vi "AutoMultiBall.vi"(8 "error in (no error)":errorcluster, 9 "Hot?":bool, 10 "Camera?":bool, 11 "ShotCount":u8=2) -> (0 "error out":errorcluster)   [LabVIEW 2013]
uses:
  AutoMultiBallStates.ctl
  ShooterStates.ctl
  <vilib>/Rock Robotics/WPI/Solenoid/WPI_SolenoidSetEnum.vi
  <vilib>/Rock Robotics/WPI/Solenoid/WPI_SolenoidValue.ctl
  Robot Global Data.vi
  ShooterCmds.ctl
  Position Typedef.ctl
panel:
  in  "Angle to Turn":dbl=15.0 format="%#_13g"
  in  "Not Hot Delay":u32=4000
  in  "Speed":dbl=0.75
  in  "Angle":dbl
  in  "Distance":dbl=84.0
  in  "Transfer Timeout (ms)":u32=1000
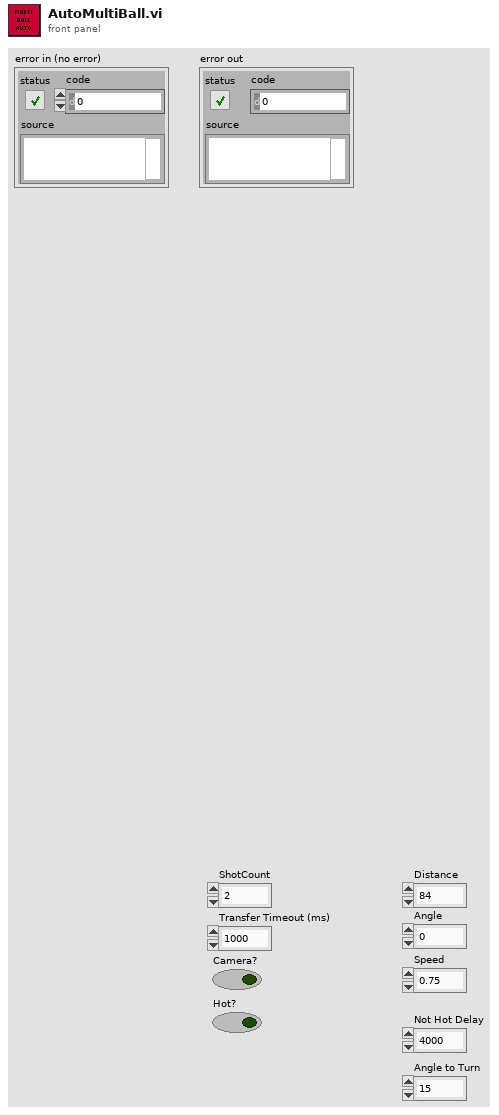
[diagram p1: front panel]
types:
  T1 = typedef "AutoMultiBallStates.ctl" = enum16{"Setup", "Wait To Fire", "Not Hot Delay", "Fire", "Pickup", "Transfer", "Cleanup"}
  T2 = typedef "WPI_SolenoidDevRef.ctl" = cluster{"DevStatus":errorcluster, "Solenoid Module":T3, "Forward Solenoid Channel":T4, "Reverse Solenoid Channel":T4}
  T3 = typedef "FPGA_TypedefSolenoidModule.ctl" = enum16{"Solenoid Module 1", "Solenoid Module 2"}
  T4 = typedef "WPI_SolenoidChannel.ctl" = enum8{"Solenoid 1", "Solenoid 2", "Solenoid 3", "Solenoid 4", "Solenoid 5", "Solenoid 6", "Solenoid 7", "Solenoid 8", "Invalid"}
  T5 = typedef "Position Typedef.ctl" = cluster{"X":dbl, "Y":dbl, "Heading":dbl}
  T6 = typedef "WPI_SolenoidValue.ctl" = enum16{"Off", "On", "Forward", "Reverse"}
  T7 = typedef "ShooterCmds.ctl" = enum16{"Fire", "Lob", "Retract", "End Of Match", "Release", "FireAuto"}
  T8 = typedef "ShooterStates.ctl" = enum16{"Init", "Ready", "RetractFull", "Disengage Clutch", "Clutch Delay", "Fire", "Fire Delay", "Latch", "Retract", "Release"}
  T9 = typedef "WPI_MotorControlDeviceRef.ctl" = cluster{"DeviceStatus":errorcluster, "Type":enum16{"PWM", "CAN"}, "PWM":cluster{"Digital Module":T10, "PWM Channel":T11, "DeadBand":T12}, "CAN":cluster{"Device Number":u8, "Control Mode":T13, "Semaphore":T14, "Max Vout":dbl}, "Invert":bool, "TransformRef":T15, "InvTransformRef":T15}
  T10 = typedef "FPGA_TypedefDigitalModule.ctl" = enum16{"Digital Module 1", "Digital Module 2"}
  T11 = typedef "FPGA_DIOPWMChannel.ctl" = enum8{"PWM 1", "PWM 2", "PWM 3", "PWM 4", "PWM 5", "PWM 6", "PWM 7", "PWM 8", "PWM 9", "PWM 10", "Invalid"}
  T12 = typedef "WPI_PWMDeadband.ctl" = cluster{"Name":string, "maxPositivePwm":i32, "minPositivePwm":i32, "centerPwm":i32, "maxNegativePwm":i32, "minNegativePwm":i32, "angularRange":u16}
  T13 = typedef "WPI_CANJaguar_ControlMode.ctl" = enum8{"Percent VBus", "Current", "Speed", "Position", "Voltage"}
  T14 = typedef "Semaphore RefNum" = refnum<k1>
  T15 = typedef "WPI_PWMTransform_ConPane.ctl" = refnum<vi>
  T16 = typedef "WPI_DigitalInputDevRef.ctl" = cluster{"DevStatus":errorcluster, "DIO Channel":T17, "Digital Module":T10}
  T17 = typedef "FPGA_DIOChannel.ctl" = enum8{"DIO 1", "DIO 2", "DIO 3", "DIO 4", "DIO 5", "DIO 6", "DIO 7", "DIO 8", "DIO 9", "DIO 10", "DIO 11", "DIO 12", "DIO 13", "DIO 14", "Invalid"}
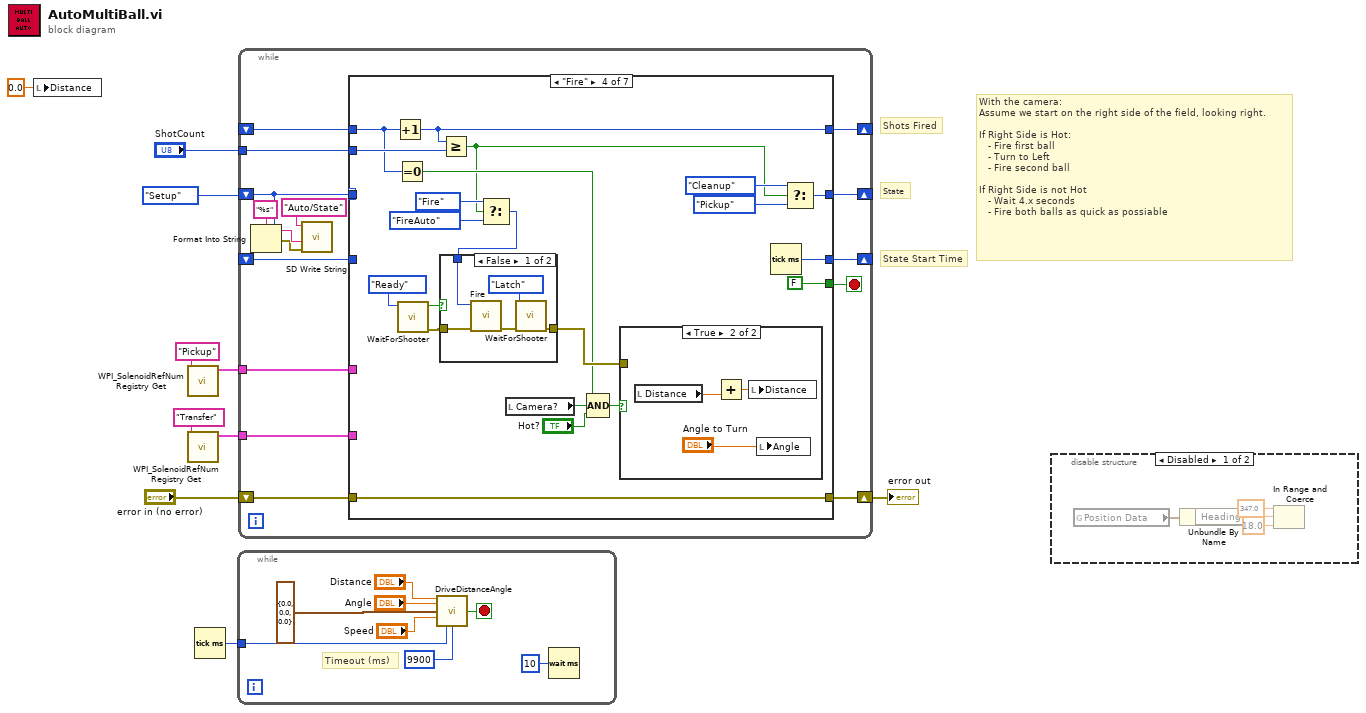
[diagram p0: block diagram]
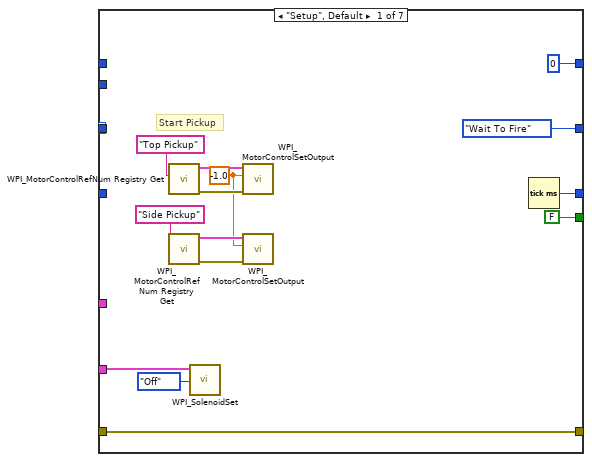
[diagram p3: hidden frame]
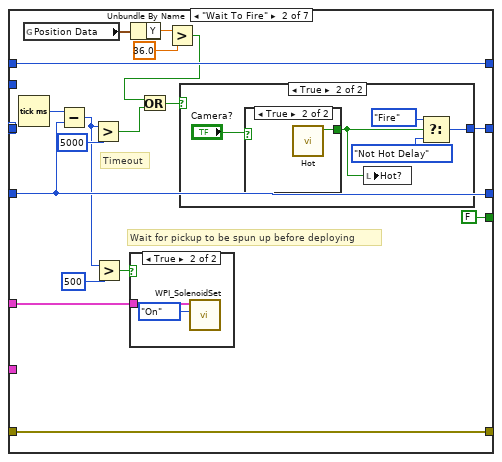
[diagram p4: hidden frame]
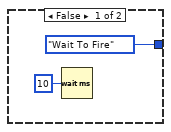
[diagram p6: hidden frame]
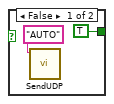
[diagram p7: hidden frame]
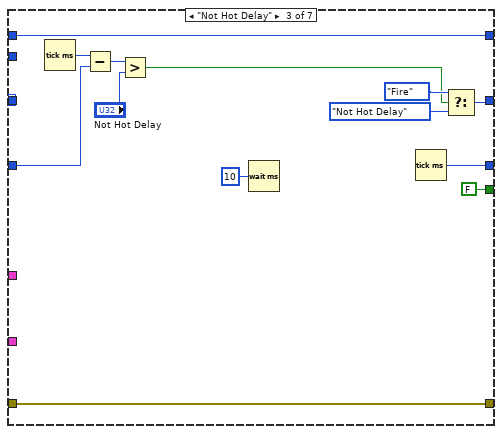
[diagram p8: hidden frame]
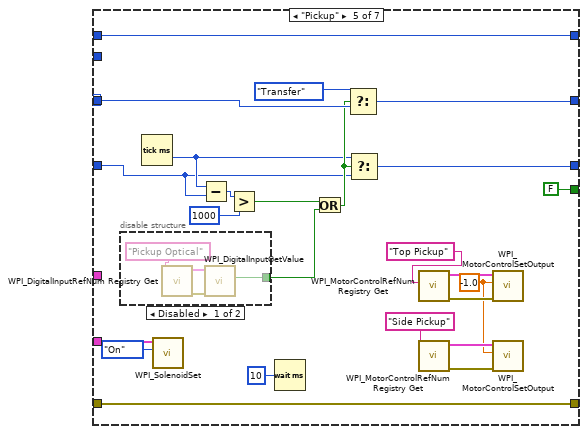
[diagram p11: hidden frame]
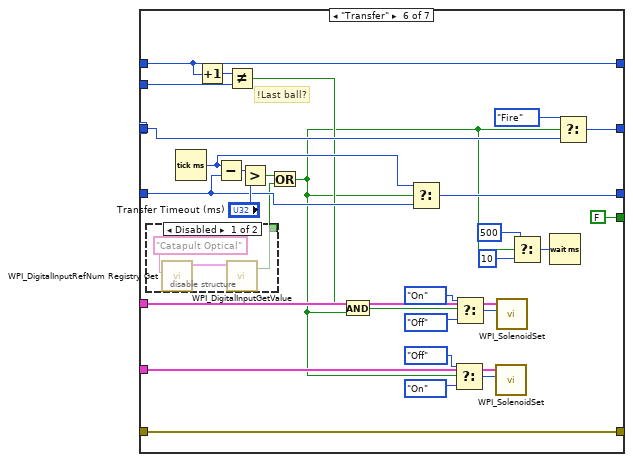
[diagram p13: hidden frame]
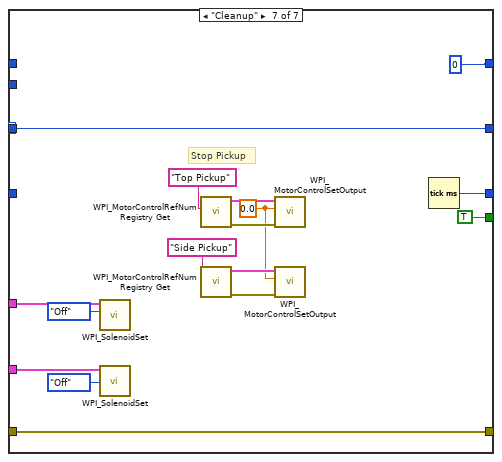
[diagram p15: hidden frame]
diagram:
  # "With the camera:\nAssume we start on the right side of the field, looking right.\n\nIf Right Side is Hot:\n   - Fire first ball\n   - Turn to Left \n   - Fire second ball\n\nIf Right Side is not Hot\n   - Wait 4.x seconds\n   - Fire both balls as quick as possiable"
  # "State Start Time"
  # "State"
  # "Shots Fired"
  n1 = local write "Distance"(0.0 ("X Target")) -> ()
  n2 = call <vilib>:"WPI_SolenoidRefNum Registry Get.vi"("refnum name"="Pickup") -> ("SolenoidDevRef"=w6:T2)  [unwired: 9 in, 1 out]
  n3 = call <vilib>:"WPI_SolenoidRefNum Registry Get.vi"("refnum name"="Transfer") -> ("SolenoidDevRef"=w4:T2)  [unwired: 9 in, 1 out]
  n4 = Tick Count (ms)() -> (millisecond timer value=w1:u32)
  n5 = while {
    tunnel: w1 -> [w17]
    stop <- w15 stop-if-true
    # "Timeout (ms)"
    n6 = call "DriveDistanceAngle.vi"("Distance"="Distance", "Angle"="Angle", "Starting Position"=T5 {"X"=0.0, "Y"=0.0, "Heading"=0.0}, "Speed"="Speed", "Start time"=w17, "Timeout (ms)"=u32 9900 ("y")) -> ("Timeout?"=w15:bool)  [unwired: 6 in, 3 out]
    n7 = Wait (ms)(milliseconds to wait=u32 10) -> ()  [unwired: 1 out]
  }
  n8 = while {
    shift-right: [w33] -> w3
    shift-left: "error in (no error)" -> [w34]
    shift-right: [w31] -> _
    shift-left: _ -> [w32]
    shift-right: [w29] -> _
    shift-left: AutoMultiBallStates."Setup" -> [w19]
    shift-right: [w27] -> _
    shift-left: _ -> [w28]
    tunnel: "ShotCount" -> [w26]
    tunnel: w6 -> [w25]
    tunnel: w4 -> [w24]
    stop <- w30 stop-if-true
    n9 = Format Into String(format string="%s", w19) -> (resulting string=w22:string, error out=w21:errorcluster)  [unwired: 2 in]
    n10 = call <vilib>:"SD Write String.vi"("error in"=w21, "String"=w22, "Name"="Auto/State") -> ()  [unwired: 7 in, 2 out]
    n11 = case shown="\"Fire\"" w19 {
      selector: w19 -> [_ _ _ _ w144 w177 _]
      tunnel: w34 -> [w35 w65 w88 w111 w142 w176 w183]
      tunnel: [w35 w65 w88 w111 w142 w176 w183] -> w33
      tunnel: [AutoMultiBallStates."Wait To Fire" w59 w79 w104 w143 w172 w182] -> w29
      tunnel: w32 -> [_ w56 w78 _ w135 w164 _]
      tunnel: [w47 w56 w87 w109 w145 w166 w196] -> w31
      tunnel: [FALSE ("At Target") FALSE ("At Target") FALSE ("At Target") FALSE FALSE FALSE ("At Target") TRUE ("At Target")] -> w30
      tunnel: w19 -> [_ _ _ _ _ _ w182]
      tunnel: w28 -> [_ w64 w90 w97 w139 w158 _]
      tunnel: [u8 0 ("ShotCount") w64 w90 w105 w139 w158 u8 0 ("ShotCount")] -> w27
      tunnel: w26 -> [_ _ _ w106 _ w156 _]
      tunnel: w25 -> [_ w58 _ _ _ w160 w193]
      tunnel: w24 -> [w37 _ _ _ w123 w168 w185]
      frame "Setup", Default {
        w38 = -1.0 ("Output")
        # "Start Pickup"
        n12 = call <vilib>:"WPI_MotorControlRefNum Registry Get.vi"("refnum name"="Top Pickup") -> ("error out"=w41:errorcluster, "MotorControlDevRef"=w45:T9)  [unwired: 9 in]
        n13 = call <vilib>:"WPI_MotorControlRefNum Registry Get.vi"("refnum name"="Side Pickup") -> ("error out"=w43:errorcluster, "MotorControlDevRef"=w42:T9)  [unwired: 9 in]
        n14 = call-poly <vilib>:"WPI_SolenoidSet.vi"("Value"=WPI_SolenoidValue."Off", "SolenoidDevRef"=w37) -> ()  [unwired: 8 in, 2 out]
        n15 = call <vilib>:"WPI_MotorControlSetOutput.vi"("error in (no error)"=w41, "Output"=w38, "MotorControlDevRef"=w45) -> ()  [unwired: 6 in, 3 out]
        n16 = call <vilib>:"WPI_MotorControlSetOutput.vi"("error in (no error)"=w43, "Output"=w38, "MotorControlDevRef"=w42) -> ()  [unwired: 6 in, 3 out]
        n17 = Tick Count (ms)() -> (millisecond timer value=w47:u32)
      }
      frame "Wait To Fire" {
        # "Timeout"
        # "Wait for pickup to be spun up before deploying"
        n18 = Tick Count (ms)() -> (millisecond timer value=w57:u32)
        n19 = global read "Robot Global Data.vi" "Position Data"() -> (w62:T5)
        n20 = Subtract(x=w57, y=w56) -> (x-y=w52:u32)
        n21 = Greater?(x=w52, y=u32 5000) -> (0:w49:bool)
        n22 = Greater?(x=w52, y=u32 500) -> (0:w54:bool)
        n23 = case shown="True" w54 {
          tunnel: w58 -> [_ w66]
          frame False {
          }
          frame True {
            n24 = call-poly <vilib>:"WPI_SolenoidSet.vi"("Value"=WPI_SolenoidValue."On", "SolenoidDevRef"=w66) -> ()  [unwired: 8 in, 2 out]
          }
        }
        n25 = Unbundle By Name(w62) -> ("Y"=w61:dbl)
        n26 = Greater?(x=w61, y=36.0) -> (0:w50:bool)
        n27 = Or(x=w50, y=w49) -> (x .or. y?=w51:bool)
        n28 = case shown="True" w51 {
          tunnel: [AutoMultiBallStates."Wait To Fire" ("f") w71] -> w59
          frame False {
            n29 = Wait (ms)(milliseconds to wait=u32 10) -> ()  [unwired: 1 out]
          }
          frame True {
            n30 = case shown="True" "Camera?" {
              tunnel: [TRUE ("Hot?") w77] -> w73
              frame False {
                n31 = call "SendUDP.vi"("data in"="AUTO") -> ()  [unwired: 10 in, 1 out]
              }
              frame True {
                n32 = call "Hot.vi"() -> ("Hot?"=w77:bool)  [unwired: 8 in, 3 out]
              }
            }
            n33 = local write "Hot?"(w73) -> ()
            n34 = Select(t=AutoMultiBallStates."Fire", s=w73, f=AutoMultiBallStates."Not Hot Delay") -> (s? t:f=w71:T1)
          }
        }
      }
      frame "Not Hot Delay" {
        n35 = Tick Count (ms)() -> (millisecond timer value=w85:u32)
        n36 = Subtract(x=w85, y=w78) -> (x-y=w84:u32)
        n37 = Greater?(x=w84, y="Not Hot Delay") -> (0:w80:bool)
        n38 = Wait (ms)(milliseconds to wait=u32 10) -> ()  [unwired: 1 out]
        n39 = Tick Count (ms)() -> (millisecond timer value=w87:u32)
        n40 = Select(t=AutoMultiBallStates."Fire", s=w80, f=AutoMultiBallStates."Not Hot Delay") -> (s? t:f=w79:T1)
      }
      frame "Fire" {
        n41 = Increment(x=w97) -> (x+1=w105:u8)
        n42 = Equal To 0?(x=w97) -> (x = 0?=w96:bool)
        n43 = call "WaitForShooter.vi"("State"=ShooterStates."Ready") -> ("error out"=w103:errorcluster, "Timeout"=w101:bool)  [unwired: 9 in]
        n44 = Greater Or Equal?(x=w105, y=w106) -> (x >= y?=w93:bool)
        n45 = Select(t=ShooterCmds."Fire", s=w93, f=ShooterCmds."FireAuto") -> (s? t:f=w92:T7)
        n46 = case shown="False" w101 {
          tunnel: w103 -> [w118 w121]
          tunnel: [w117 w121] -> w98
          tunnel: w92 -> [w116 _]
          frame False {
            n47 = call "Fire.vi"("error in (no error)"=w118, 11:w116) -> ("error out"=w119:errorcluster)  [unwired: 9 in]
            n48 = call "WaitForShooter.vi"("error in (no error)"=w119, "State"=ShooterStates."Latch") -> ("error out"=w117:errorcluster)  [unwired: 8 in, 1 out]
          }
          frame True {
          }
        }
        n49 = local read "Camera?"() -> (w100:bool)
        n50 = Compound Arithmetic op=AND(w96, w100, "Hot?") -> (w99:bool)
        n51 = case shown="True" w99 {
          tunnel: w98 -> [_ _]
          frame False {
          }
          frame True {
            n52 = local read "Distance"() -> (w115:dbl)
            n53 = Add(y=w115) -> (x=w113:dbl, x+y=w114:dbl)
            n54 = local write "Distance"(w114) -> ()
            n55 = local write "Angle"("Angle to Turn") -> ()
          }
        }
        n56 = Tick Count (ms)() -> (millisecond timer value=w109:u32)
        n57 = Select(t=AutoMultiBallStates."Cleanup", s=w93, f=AutoMultiBallStates."Pickup") -> (s? t:f=w104:T1)
      }
      frame "Pickup" {
        w124 = -1.0 ("Output")
        n58 = disable-structure shown="Disabled" {
          disable-tunnel: [w146 _] -> w138
          frame Disabled {
            n59 = call <vilib>:"WPI_DigitalInputRefNum Registry Get.vi"("refnum name"="Pickup Optical") -> ("error out"=w148:errorcluster, "DigitalInputDevRef"=w147:T16)  [unwired: 9 in]
            n60 = call <vilib>:"WPI_DigitalInputGetValue.vi"("error in (no error)"=w148, "DigitalInputDevRef"=w147) -> ("Value"=w146:bool)  [unwired: 7 in, 2 out]
          }
          frame Enabled {
          }
        }
        n61 = Tick Count (ms)() -> (millisecond timer value=w136:u32)
        n62 = call-poly <vilib>:"WPI_SolenoidSet.vi"("Value"=WPI_SolenoidValue."On", "SolenoidDevRef"=w123) -> ()  [unwired: 8 in, 2 out]
        n63 = Subtract(x=w136, y=w135) -> (x-y=w134:u32)
        n64 = Greater?(x=w134, y=u32 1000) -> (0:w132:bool)
        n65 = Wait (ms)(milliseconds to wait=u32 10) -> ()  [unwired: 1 out]
        n66 = Or(x=w132, y=w138) -> (x .or. y?=w137:bool)
        n67 = Select(t=AutoMultiBallStates."Transfer", s=w137, f=w144) -> (s? t:f=w143:T1)
        n68 = Select(t=w136, s=w137, f=w135) -> (s? t:f=w145:u32)
        n69 = call <vilib>:"WPI_MotorControlRefNum Registry Get.vi"("refnum name"="Top Pickup") -> ("error out"=w126:errorcluster, "MotorControlDevRef"=w130:T9)  [unwired: 9 in]
        n70 = call <vilib>:"WPI_MotorControlRefNum Registry Get.vi"("refnum name"="Side Pickup") -> ("error out"=w128:errorcluster, "MotorControlDevRef"=w127:T9)  [unwired: 9 in]
        n71 = call <vilib>:"WPI_MotorControlSetOutput.vi"("error in (no error)"=w126, "Output"=w124, "MotorControlDevRef"=w130) -> ()  [unwired: 6 in, 3 out]
        n72 = call <vilib>:"WPI_MotorControlSetOutput.vi"("error in (no error)"=w128, "Output"=w124, "MotorControlDevRef"=w127) -> ()  [unwired: 6 in, 3 out]
      }
      frame "Transfer" {
        # "!Last ball?"
        n73 = disable-structure shown="Disabled" {
          disable-tunnel: [w181 _] -> w159
          frame Disabled {
            n74 = call <vilib>:"WPI_DigitalInputRefNum Registry Get.vi"("refnum name"="Catapult Optical") -> ("DigitalInputDevRef"=w179:T16)  [unwired: 9 in, 1 out]
            n75 = call <vilib>:"WPI_DigitalInputGetValue.vi"("DigitalInputDevRef"=w179) -> ("Value"=w181:bool)  [unwired: 8 in, 2 out]
          }
          frame Enabled {
          }
        }
        n76 = Tick Count (ms)() -> (millisecond timer value=w165:u32)
        n77 = Increment(x=w158) -> (x+1=w157:u8)
        n78 = Subtract(x=w165, y=w164) -> (x-y=w175:u32)
        n79 = Not Equal?(x=w157, y=w156) -> (x != y?=w154:bool)
        n80 = Greater?(x=w175, y="Transfer Timeout (ms)") -> (0:w167:bool)
        n81 = Or(x=w167, y=w159) -> (x .or. y?=w153:bool)
        n82 = And(x=w154, y=w153) -> (x .and. y?=w155:bool)
        n83 = Select(t=w165, s=w153, f=w164) -> (s? t:f=w166:u32)
        n84 = Select(t=WPI_SolenoidValue."Off" ("Value"), s=w153, f=WPI_SolenoidValue."On") -> (s? t:f=w171:T6)
        n85 = Select(t=WPI_SolenoidValue."On" ("Value"), s=w155, f=WPI_SolenoidValue."Off") -> (s? t:f=w163:T6)
        n86 = call-poly <vilib>:"WPI_SolenoidSet.vi"("Value"=w171, "SolenoidDevRef"=w168) -> ()  [unwired: 8 in, 2 out]
        n87 = call-poly <vilib>:"WPI_SolenoidSet.vi"("Value"=w163, "SolenoidDevRef"=w160) -> ()  [unwired: 8 in, 2 out]
        n88 = Select(t=u32 500 ("milliseconds to wait"), s=w153, f=u32 10) -> (s? t:f=w151:u32)
        n89 = Wait (ms)(milliseconds to wait=w151) -> ()  [unwired: 1 out]
        n90 = Select(t=AutoMultiBallStates."Fire", s=w153, f=w177) -> (s? t:f=w172:T1)
      }
      frame "Cleanup" {
        w186 = 0.0 ("Output")
        # "Stop Pickup"
        n91 = call-poly <vilib>:"WPI_SolenoidSet.vi"("Value"=WPI_SolenoidValue."Off", "SolenoidDevRef"=w193) -> ()  [unwired: 8 in, 2 out]
        n92 = call-poly <vilib>:"WPI_SolenoidSet.vi"("Value"=WPI_SolenoidValue."Off", "SolenoidDevRef"=w185) -> ()  [unwired: 8 in, 2 out]
        n93 = call <vilib>:"WPI_MotorControlRefNum Registry Get.vi"("refnum name"="Top Pickup") -> ("error out"=w188:errorcluster, "MotorControlDevRef"=w192:T9)  [unwired: 9 in]
        n94 = call <vilib>:"WPI_MotorControlRefNum Registry Get.vi"("refnum name"="Side Pickup") -> ("error out"=w190:errorcluster, "MotorControlDevRef"=w189:T9)  [unwired: 9 in]
        n95 = call <vilib>:"WPI_MotorControlSetOutput.vi"("error in (no error)"=w188, "Output"=w186, "MotorControlDevRef"=w192) -> ()  [unwired: 6 in, 3 out]
        n96 = call <vilib>:"WPI_MotorControlSetOutput.vi"("error in (no error)"=w190, "Output"=w186, "MotorControlDevRef"=w189) -> ()  [unwired: 6 in, 3 out]
        n97 = Tick Count (ms)() -> (millisecond timer value=w196:u32)
      }
    }
  }
  "error out" <- w3
  n98 = disable-structure shown="Disabled" {
    frame Disabled {
      n99 = global read "Robot Global Data.vi" "Position Data"() -> (w201:T5)
      n100 = Unbundle By Name(w201) -> ("Heading"=w200:dbl)
      n101 = In Range and Coerce(upper limit=347.0, x=w200, lower limit=18.0) -> ()  [unwired: 2 out]
    }
    frame Enabled {
    }
  }
